vi "DSF.Shared.Configuration.Execution Timing.Get Decimation.vi"(8 "error in (no error)":errorcluster, 11 "DSF.Shared.Configuration.Execution Timing in":refnum<class "DSF.Engine.Timing.lvclass">) -> (0 "error out":errorcluster, 2 "Decimation":T1=1, 3 "DSF.Shared.Configuration.Execution Timing out":refnum<class "DSF.Engine.Timing.lvclass">)   [LabVIEW 2016, in "DSF.Engine.lvlib" / "DSF.Engine.Timing.lvclass"]
uses:
  DSF.Engine.Timing.lvclass
  Shared/Typedefs/DSF.Shared.Typedefs.Scalars.Decimation.ctl
  DSF.Engine.Timing.lvclass/DSF.Engine.Timing.ctl
  DSF.Shared.lvlib
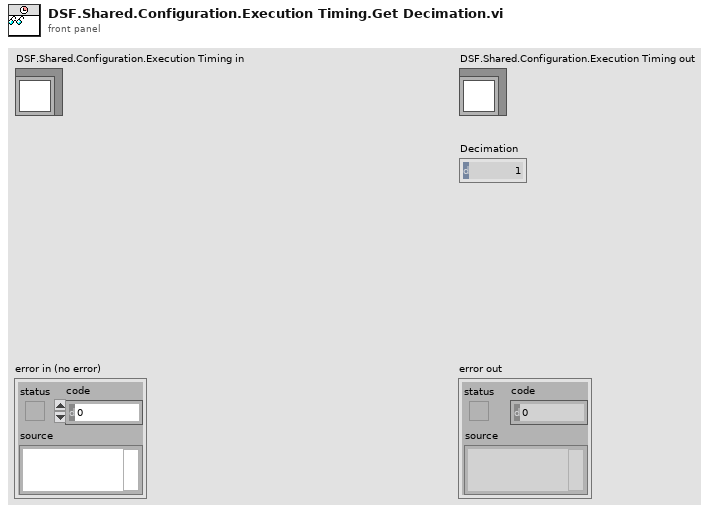
[diagram p1: front panel]
types:
  T1 = typedef "DSF.Shared.lvlib/DSF.Shared.Typedefs.Scalars.Decimation.ctl" = u64
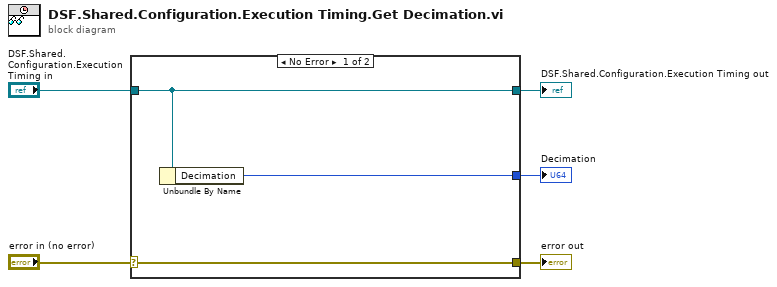
[diagram p0: block diagram]
diagram:
  n1 = case shown="No Error" "error in (no error)" {
    selector: "error in (no error)" -> [w8 w9]
    tunnel: [w8 w9] -> w4
    tunnel: [w7 w10] -> w2
    tunnel: "DSF.Shared.Configuration.Execution Timing in" -> [w7 w10]
    tunnel: [w6 _] -> w1
    frame No Error {
      n2 = Unbundle By Name(w7) -> ("Decimation"=w6:T1)
    }
    frame Error {
    }
  }
  "error out" <- w4
  "DSF.Shared.Configuration.Execution Timing out" <- w2
  "Decimation" <- w1
